vi "Max Fehler.vi"(11 "Tabelle":string[](array[string])) -> (3 "max Fehler":dbl)   [LabVIEW 2020, in "EPA 1065.lvlib" / "HovaCAL Interference verificaton.lvlib"]
uses:
  HovaCAL Interference verificaton.lvlib
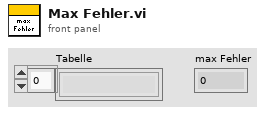
[diagram p1: front panel]
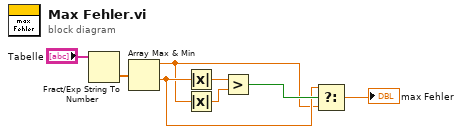
[diagram p0: block diagram]
diagram:
  n1 = Fract/Exp String To Number(string="Tabelle") -> (number=w8:dbl[])  [unwired: 3 in, 1 out]
  n2 = Array Max & Min(array=w8) -> (max value=w2:dbl, min value=w3:dbl)  [unwired: 2 out]
  n3 = Absolute Value(x=w3) -> (abs(x)=w6:dbl)
  n4 = Absolute Value(x=w2) -> (abs(x)=w5:dbl)
  n5 = Greater?(x=w6, y=w5) -> (0:w4:bool)
  n6 = Select(t=w3, s=w4, f=w2) -> (s? t:f=→"max Fehler":dbl)
